vi "Abort.vi"(0 "reference in":refnum<class "DUT_Handler_Simple.lvclass">, 5 "error in (no error)":errorcluster) -> (14 "reference in":refnum<class "DUT_Handler_Simple.lvclass">, 19 "error out":errorcluster)   [LabVIEW 2022 SP3, in "DUT_Handler_Simple.lvlib" / "DUT_Handler_Simple.lvclass"]
uses:
  DUT_Handler_Simple.lvclass
  Components/DUT_Handler_Base.lvlibp/EventData.ctl
  Components/DUT_Handler_Base.lvlibp/DUT_Handler_Base.lvclass
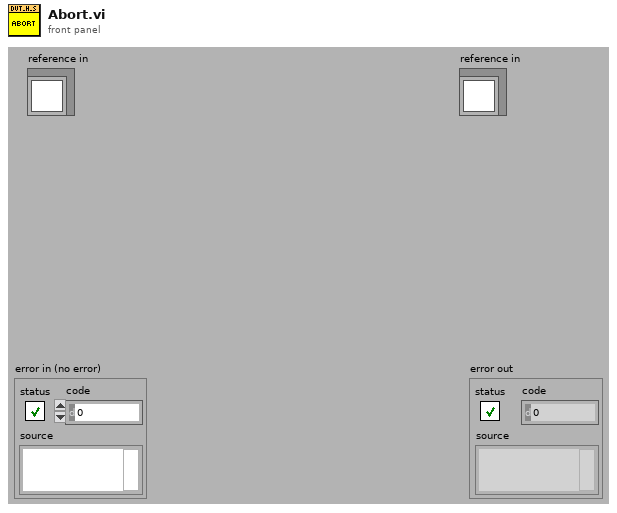
[diagram p1: front panel]
types:
  T1 = typedef "DUT_Handler_Base.lvlibp/DUT_Handler_Base.lvclass/EventData.ctl" = cluster{"Action":enum16{"Load", "Cancel", "MoveIn", "MoveOut", "Abort", "Msg", "Enabled", "Disabled", "Fault", "Shutdown"}, "SN":string, "BN":string, "DUT__ID":u32, "Message":string, "From":string, "To":string}
  T2 = enum16{"Load", "Cancel", "MoveIn", "MoveOut", "Abort", "Msg", "Enabled", "Disabled", "Fault", "Shutdown"}
  T3 = typedef "DUT_Handler_Simple.lvlib/DUT_Handler_Simple.lvclass/ObjectAttributes.ctl" = cluster{"Config":T4, "event_data":T1, "Enabled":bool, "Barcode_Reader":refnum<class "Barcode_Reader_Base.lvclass">}
  T4 = typedef "DUT_Handler_Simple.lvlib/DUT_Handler_Simple.lvclass/Config.ctl" = cluster{"default":string}
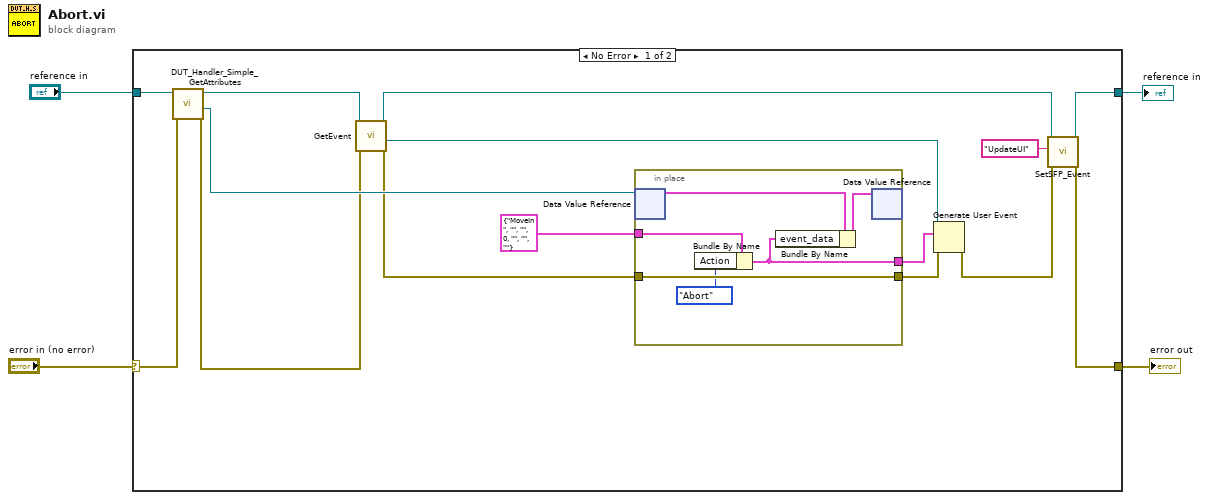
[diagram p0: block diagram]
diagram:
  n1 = case shown="No Error" "error in (no error)" {
    selector: "error in (no error)" -> [w19 w27]
    tunnel: [w12 w27] -> w2
    tunnel: [w13 w26] -> w1
    tunnel: "reference in" -> [w18 w26]
    frame No Error {
      n2 = call "DUT_Handler_Simple_GetAttributes.vi"("error in (no error)"=w19, "reference in"=w18) -> ("error out"=w10:errorcluster, "DataRef"=w15:refnum<data-value>, "reference out"=w17:refnum<class "DUT_Handler_Simple.lvclass">)  [unwired: 6 in, 1 out]
      n3 = call-dynamic "GetEvent.vi"("error in (no error)"=w10, "reference in"=w17) -> ("error out"=w8:errorcluster, "DUT_Handler"=w16:refnum<user-event>, "reference in"=w14:refnum<class "DUT_Handler_Simple.lvclass">)  [unwired: 6 in]
      n4 = in-place {
        in-place-border: [w23] -> w6
        in-place-border: w8 -> [w23]
        in-place-border: T1 {"Action"=enum."MoveIn", "SN"="", "BN"="", "DUT__ID"=0, "Message"="", "From"="", "To"=""} ("event_data") -> [w22]
        in-place-border: [w20] -> w5
        n5 = in-place-dvr #1(w15) -> (w25:T3)  [unwired: 1 out]
        n6 = Bundle By Name(cluster=w22, "Action"=T2."Abort") -> (w20:T1)
        n7 = Bundle By Name(cluster=w25, "event_data"=w20) -> (w24:T3)
        n8 = in-place-dvr #1(w24) -> ()  [unwired: 2 out]
      }
      n9 = Generate User Event(user event=w16, event data cluster=w5, error in=w6) -> (error out=w7:errorcluster)  [unwired: 1 in, 1 out]
      n10 = call-dynamic "SetSFP_Event.vi"("error in (no error)"=w7, "msg"="UpdateUI", "reference in"=w14) -> ("error out"=w12:errorcluster, "reference out"=w13:refnum<class "DUT_Handler_Simple.lvclass">)  [unwired: 7 in]
    }
    frame Error {
    }
  }
  "error out" <- w2
  "reference in" <- w1
